vi "Get Image Descriptor.vi"(8 "error in (no error)":errorcluster caption="错误输入（无错误）", 11 "Gif Image 输入":refnum<class "Gif Image.lvclass"> caption="DNL_LabVIEW Object in") -> (0 "error out":errorcluster caption="错误输出", 2 "Image Descriptor":T1 {"Image ID" format="%02x"}, 3 "Gif Image 输出":refnum<class "Gif Image.lvclass"> caption="DNL_LabVIEW Object out")   [LabVIEW 2012, in "Picture Box Tools.lvlib" / "Gif Image.lvclass"]
uses:
  Gif Image.lvclass
  Control/Image Descriptor.ctl
  Control/ID Charactor.ctl
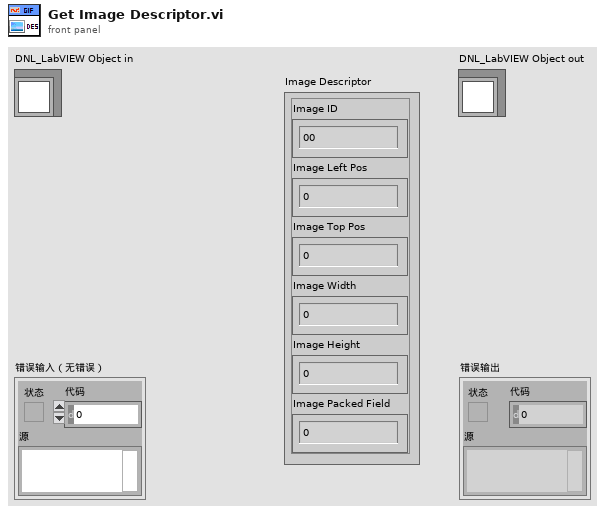
[diagram p1: front panel]
types:
  T1 = typedef "Picture Box Tools.lvlib/Gif Image.lvclass/Image Descriptor.ctl" = cluster{"Image ID":u8, "Image Left Pos":u16, "Image Top Pos":u16, "Image Width":u16, "Image Height":u16, "Image Packed Field":u8}
  T2 = enum16{"big-endian, network order", "native, host order", "little-endian"}
  T3 = typedef "Picture Box Tools.lvlib/Gif Image.lvclass/ID Charactor.ctl" = u8
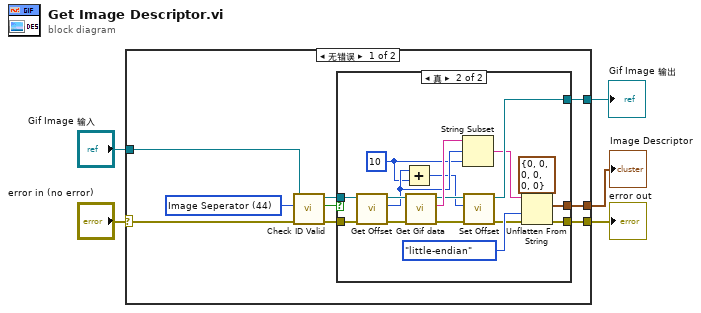
[diagram p0: block diagram]
diagram:
  n1 = case shown="无错误" "error in (no error)" {
    selector: "error in (no error)" -> [w13 w35]
    tunnel: [w7 w35] -> w4
    tunnel: [w9 w34] -> w2
    tunnel: "Gif Image 输入" -> [w14 w34]
    tunnel: [w6 _] -> w1
    frame No Error {
      w12 = T3 44 items=["Image Seperator"=44, "Extension Introducer"=33, "Graphic Control Label"=249, "Comment Label"=254, "PlainText Label"=1, "Gif Trailor"=59, "Application Label"=255] ("ID")
      n2 = call "Check ID Valid.vi"("error in (no error)"=w13, "ID"=w12, "Gif Image 输入"=w14) -> ("error out"=w8:errorcluster, "ID Valid"=w11:bool, "Gif Image 输出"=w10:refnum<class "Gif Image.lvclass">)  [unwired: 5 in, 1 out]
      n3 = case shown="真" w11 {
        tunnel: w10 -> [w16 w33]
        tunnel: [w16 w23] -> w9
        tunnel: w8 -> [w15 w31]
        tunnel: [w15 w17] -> w7
        tunnel: [_ w19] -> w6
        frame False {
        }
        frame True {
          w27 = 10 ("长度（剩余）")
          n4 = call "Get Offset.vi"("error in (no error)"=w31, "Gif Image输入"=w33) -> ("error out"=w30:errorcluster, "Offset"=w28:i32, "Gif Image输出"=w32:refnum<class "Gif Image.lvclass">)  [unwired: 7 in]
          n5 = Add(x=w28, y=w27) -> (x+y=w24:i32)
          n6 = call "Get Gif data.vi"("error in (no error)"=w30, "Gif Image输入"=w32) -> ("error out"=w25:errorcluster, "Gif data"=w29:string, "Gif Image输出"=w26:refnum<class "Gif Image.lvclass">)  [unwired: 7 in]
          n7 = String Subset(string=w29, offset (0)=w28, length (rest)=w27) -> (substring=w21:string)
          n8 = call "Set Offset.vi"("error in (no error)"=w25, "Offset"=w24, "Gif Image输入"=w26) -> ("error out"=w18:errorcluster, "Gif Image输出"=w23:refnum<class "Gif Image.lvclass">)  [unwired: 7 in]
          n9 = Unflatten From String(type=T1 {"Image ID"=0, "Image Left Pos"=0, "Image Top Pos"=0, "Image Width"=0, "Image Height"=0, "Image Packed Field"=0} ("Image Descriptor"), binary string=w21, byte order (0:big-endian, network order)=T2."little-endian" ("字节顺序(0:big-endian, network order)"), error in (no error)=w18) -> (value=w19:T1, error out=w17:errorcluster)  [unwired: 1 in, 1 out]
        }
      }
    }
    frame Error {
    }
  }
  "error out" <- w4
  "Gif Image 输出" <- w2
  "Image Descriptor" <- w1
